vi "Convert Message.vi"(8 "error in (no error)":errorcluster, 11 "Throttle Position in":refnum<class "Throttle Position.lvclass">) -> (0 "error out":errorcluster, 1 "variant":variant, 2 "Result":dbl, 3 "Throttle Position out":refnum<class "Throttle Position.lvclass">)   [LabVIEW 2011, in "Throttle Position.lvclass"]
uses:
  Throttle Position.lvclass
  PID.lvclass
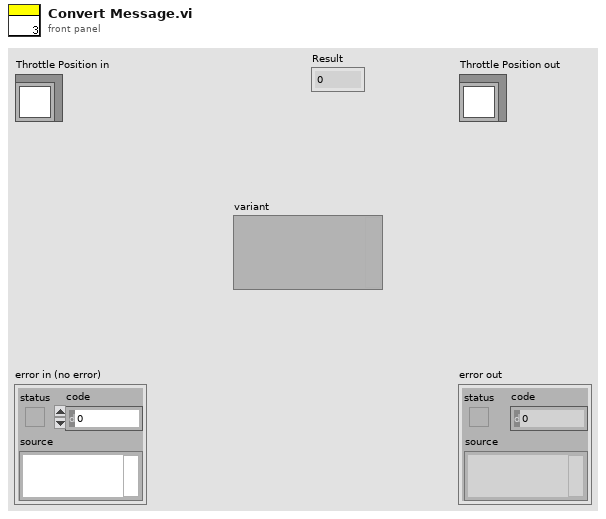
[diagram p1: front panel]
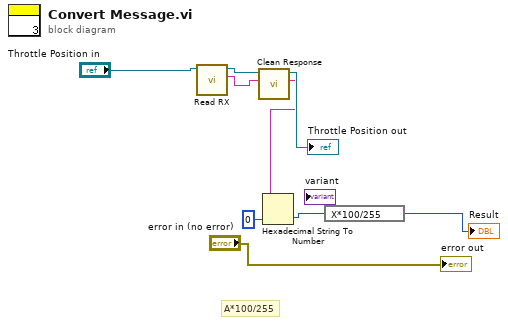
[diagram p0: block diagram]
diagram:
  # "A*100/255"
  n1 = call "Read RX.vi"("PID in"="Throttle Position in") -> ("RX"=w1:string, "PID out"=w2:refnum<class "Throttle Position.lvclass">)  [unwired: 8 in, 1 out]
  n2 = call-dynamic "Clean Response.vi"("Response In"=w1, "PID.lvclass"=w2) -> ("result string"=w4:string, "PID.lvclass 2"=→"Throttle Position out":refnum<class "Throttle Position.lvclass">)  [unwired: 7 in, 1 out]
  n3 = Hexadecimal String To Number(string=w4, default (0uL)=u8 0 ("default (0 U32)")) -> (number=w8:u8)  [unwired: 1 in, 1 out]
  n4 = expression code="X*100/255"(w8) -> (→"Result":u8)
  "error out" <- "error in (no error)"
